vi "Read UI VI.vi"(8 "error in (no error)":errorcluster, 11 "UI CMD in":refnum<class "UI CMD.lvclass">) -> (0 "error out":errorcluster, 2 "UI VI":refnum<vi>, 3 "UI CMD out":refnum<class "UI CMD.lvclass">)   [LabVIEW 2014, in "UI CMD.lvclass"]
uses:
  UI CMD.lvclass
  UI CMD.lvclass/UI CMD.ctl
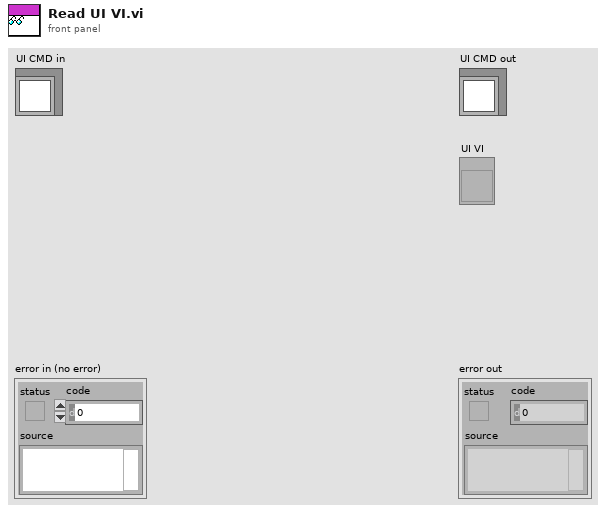
[diagram p1: front panel]
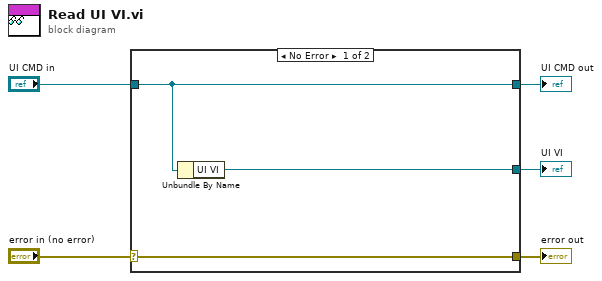
[diagram p0: block diagram]
diagram:
  n1 = case shown="No Error" "error in (no error)" {
    selector: "error in (no error)" -> [w8 w9]
    tunnel: [w8 w9] -> w4
    tunnel: [w7 w10] -> w2
    tunnel: "UI CMD in" -> [w7 w10]
    tunnel: [w6 _] -> w1
    frame No Error {
      n2 = Unbundle By Name(w7) -> ("UI VI"=w6:refnum<vi>)
    }
    frame Error {
    }
  }
  "error out" <- w4
  "UI CMD out" <- w2
  "UI VI" <- w1
